vi "WF phase diversity_MATLAB_Correction_loop_AndorSDK_OneCorrApplyToAll.vi"() -> ()   [LabVIEW 2018]
uses:
  <userlib>/WaveKit.lib/Controls/Wavefront Corrector states - ONE.ctl
  <userlib>/WaveKit.lib/Classes/WavefrontCorrector/WavefrontCorrector.lvclass
  <userlib>/WaveKit.lib/Classes/WavefrontCorrectorSet/WavefrontCorrectorSet.lvclass
  <vilib>/Analysis/1siggen.llb/Ramp Pattern by Samples.vi
  <vilib>/Utility/file.llb/Read From Spreadsheet File (DBL).vi
  <vilib>/Analysis/1siggen.llb/Ramp Pattern by Delta.vi
  <vilib>/Analysis/NI_AALBase.lvlib
panel:
  in  "Tab Control":T1(tab)
  in  "Offset command file":path=path "D:/SystemAlignment/system_aberration_20200206.dat"
  in  "Initial haso file":path=path "D:/SystemAlignment/system_aberration_residual_20191015.has"
  out "# of Phase":i32
  in  "Error in":errorcluster
  in  "DM configuration file":path=path "C:/Program Files (x86)/Imagine Optic/Configuration Files/WaveFrontCorrector_mirao52-e_0326.dat"
  out "DM Initial State":T2[](array[typedef])
  out "DM ActuatorsNumber":i32
  out "Error out":errorcluster
  in  "EMCCD trigger port":tag="Dev1/port0/line0"
  in  "Cooler set to Temperature":i32=-60
  in  "Trigger":u32(ring)=1 items=["Internal", "External"]
  out "Return from CheckTimings":u32
  out "Calculated Exposure Value":sgl format="%.2f"
  out "Return from SetTemperature":u32
  out "Cooling":i32
  out "Return from Initialize":u32
  out "Detector X Pixels":i32
  out "Detector Y Pixels":i32
  in  "Initialize EMCCD?":bool=TRUE
  in  "Turn off EMCCD when finished?":bool=TRUE
  in  "Initial Zer coeff":dbl[](array[numeric])=[0.2, 0.2]
  in  "Initial Zer index":dbl[](array[numeric])=[4.0, 5.0]
  out "Initial Zer coeff\nRandomly generated":dbl[](array[numeric])
  out "Initial Zer index (starting from 4)\nrandomly generated":dbl[](array[numeric])
  in  "aberration tolerance":dbl=0.1 format="%#_13g"
  in  "aberration threshold":dbl=0.25 format="%#_13g"
  in  "?":enum16{"input manually ", "randomly generated"}(ring)
  in  "max random order":i64=9
  in  "NOT YET: Data Acquisition Iteration #":i32=1
  in  "Zern index in 2":i32[](array[numeric])=[3, 4, 5, 6, 7, 8]
  in  "Zern coef in 2":sgl[](array[numeric])=[0.0, 0.0, 0.2, 0.0, 0.0, 0.0]
  in  "Zern index in 3":i32[](array[numeric])=[3, 4, 5, 6, 7, 8]
  in  "Zern coef in 3":sgl[](array[numeric])=[0.2, 0.0, 0.0, 0.0, 0.0, 0.0]
  in  "Zern index in 4":i32[](array[numeric])=[3, 4, 5, 6, 7, 8]
  in  "Zern coef in 4":sgl[](array[numeric])=[0.2, 0.0, 0.0, 0.0, 0.0, 0.0]
  in  "Zern index in 5":i32[](array[numeric])=[3, 4, 5, 6, 7, 8]
  in  "Zern coef in 5":sgl[](array[numeric])=[0.0, 0.0, 0.0, 0.0, 0.0, -0.2]
  in  "Andor Picture/notes save to path":path=path "D:/YD/test/test1"
  in  "base name":string="beads_test"
  in  "Pics/phase":dbl=2.0
  in  "camera exposure time (s)":string="0.02"
  in  "# of Phase":i32=5
  in  "COMMAND matrix path":path=path "D:/SystemAlignment/IM_20200224.aomi"
  in  "488 shutter":refnum<k7>(container)
  in  "?":bool
  out "phase diversity file name":string
  out "Corrected Picture name":string
  in  "Z for correction (um) (10 steps=1um)":dbl format="%#_13g"
  in  "ASI stage VISA resource name":refnum<visa-resource-name>="COM5"
  in  "Z scanning range (um)":dbl format="%#_13g"
  in  "Z scanning step (um)":dbl format="%#_13g"
  out "Current Z in step":string="where z"
  in  "Use GPU":bool=TRUE
  in  "Show Recon":bool=TRUE
  in  "Show Input":bool
  in  "Background Value":u32=290
  in  "Crop Size of image":u32=512
  in  "Gamma Value":dbl=1e-06
  in  "Iteration Number":u32=10
  in  "Zernike Order":u32=15
  in  "Number for average":u32=2
  in  "Number of Phase":u32=2
  in  "Run MATLAB or correction?":bool=TRUE
  in  "Keep Reconstructed Defocus component?":bool
  # "If Pics/phase is 2:\npicture order:\n\noffset+aberr *2\nphase diversity *8\n\nground truth *1\noffset+aberr *1\ncorrected *2 but the last one cannot be seen in imagej"
  # "Randomly Generate Initial Zernike, enter here:"
  # "Manually input, enter here:"
  # "Andor Camera Settings"
  # "z-stack is from (Z_for_correction-Z_scanning_range) to (Z_for_correction+Z_scanning_range)"
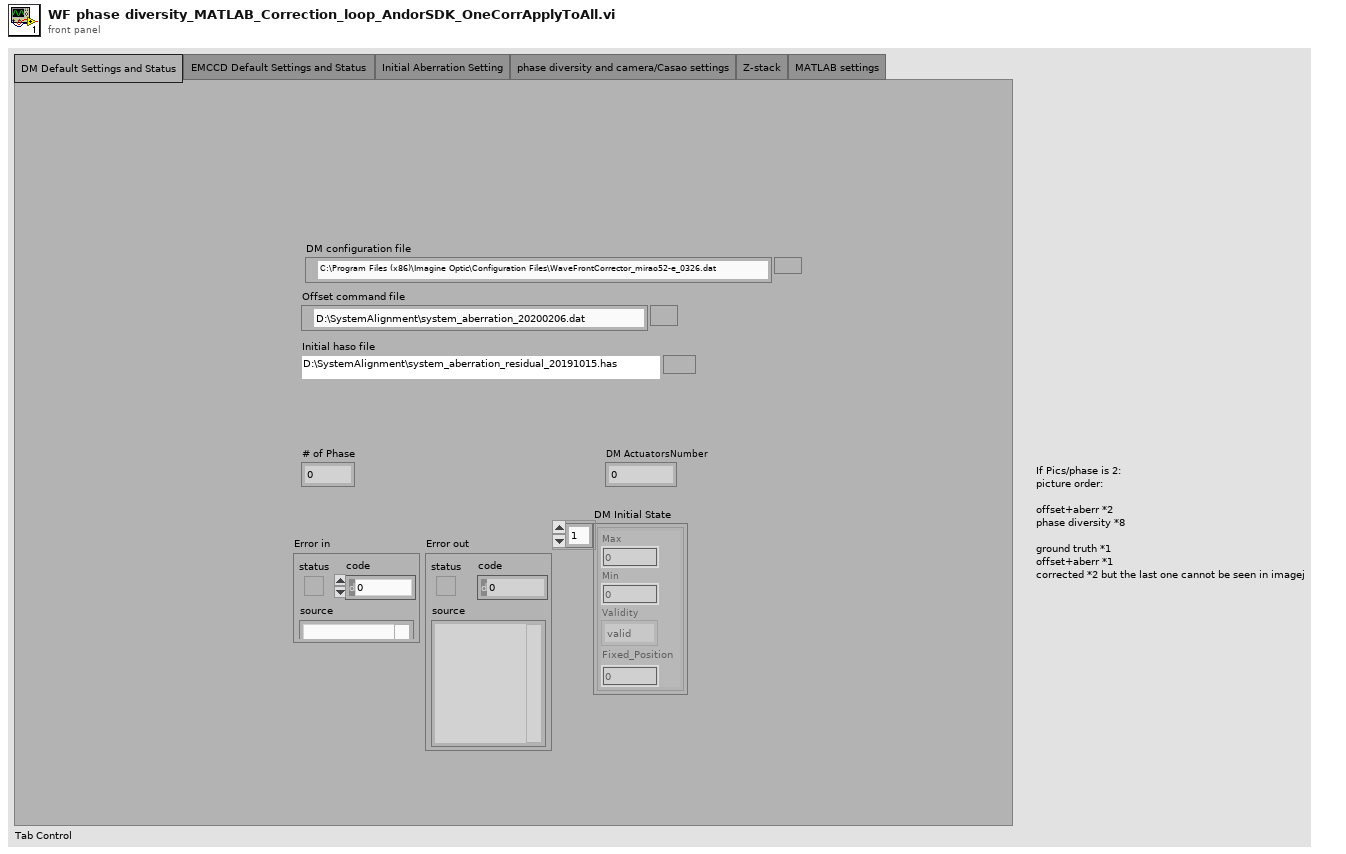
[diagram p1: front panel]
types:
  T1 = enum32{"DM Default Settings and Status", "EMCCD Default Settings and Status ", "Initial Aberration Setting", "phase diversity and camera/Casao settings", "Z-stack", "MATLAB settings"}
  T2 = typedef "Wavefront Corrector states - ONE.ctl" = cluster{"Max":sgl, "Min":sgl, "Validity":enum16{"valid", "fixed", "invalid"}, "Fixed_Position":sgl}
  T3 = typedef "Error Code Enum typedef.ctl" = enum32{"N/A (0)", "DRV_ERROR_CODES", "DRV_SUCCESS", "DRV_VXDNOTINSTALLED", "DRV_ERROR_SCAN", "DRV_ERROR_CHECK_SUM", "DRV_ERROR_FILELOAD", "DRV_UNKNOWN_FUNC", "DRV_ERROR_VXD_INIT", "DRV_ERROR_ADDRESS", "DRV_ERROR_PAGELOCK", "DRV_ERROR_PAGEUNLOCK", "DRV_ERROR_BOARDTEST", "DRV_ERROR_ACK", "DRV_ERROR_UP_FIFO", "DRV_ERROR_PATTERN", "N/A (16)", "DRV_ACQUISITION_ERRORS", "DRV_ACQ_BUFFER", "DRV_ACQ_DOWNFIFO_FULL", "DRV_PROC_UNKONWN_INSTRUCTION", "DRV_ILLEGAL_OP_CODE", "DRV_KINETIC_TIME_NOT_MET", "DRV_ACCUM_TIME_NOT_MET", "DRV_NO_NEW_DATA", "N/A (25)", "DRV_SPOOLERROR", "N/A (27)", "N/A (28)", "N/A (29)", "N/A (30)", "N/A (31)", "N/A (32)", "DRV_TEMPERATURE_CODES", "DRV_TEMPERATURE_OFF", "DRV_TEMPERATURE_NOT_STABILIZED", "DRV_TEMPERATURE_STABILIZED", "DRV_TEMPERATURE_NOT_REACHED", "DRV_TEMPERATURE_OUT_RANGE", "DRV_TEMPERATURE_NOT_SUPPORTED", "DRV_TEMPERATURE_DRIFT", "N/A (41)", "N/A (42)", "N/A (43)", "N/A (44)", "N/A (45)", "N/A (46)", "N/A (47)", "N/A (48)", "DRV_GENERAL_ERRORS", "DRV_INVALID_AUX", "DRV_COF_NOTLOADED", "DRV_FPGAPROG", "DRV_FLEXERROR", "DRV_GPIBERROR", "N/A (55)", "N/A (56)", "N/A (57)", "N/A (58)", "N/A (59)", "N/A (60)", "N/A (61)", "N/A (62)", "N/A (63)", "DRV_DATATYPE", "DRV_DRIVER_ERRORS", "DRV_P1INVALID", "DRV_P2INVALID", "DRV_P3INVALID", "DRV_P4INVALID", "DRV_INIERROR", "DRV_COFERROR", "DRV_ACQUIRING", "DRV_IDLE", "DRV_TEMPCYCLE", "DRV_NOT_INITIALIZED", "DRV_P5INVALID", "DRV_P6INVALID", "DRV_INVALID_MODE", "DRV_INVALID_FILTER", "DRV_I2CERRORS", "DRV_I2CDEVNOTFOUND", "DRV_I2CTIMEOUT", "DRV_P7INVALID", "N/A (84)", "N/A (85)", "N/A (86)", "N/A (87)", "N/A (88)", "N/A (89)", "DRV_IOCERROR", "DRV_VRMVERSIONERROR"}
  T4 = typedef "NI_Matrix.lvlib/RealMatrix.ctl" = dbl[][]
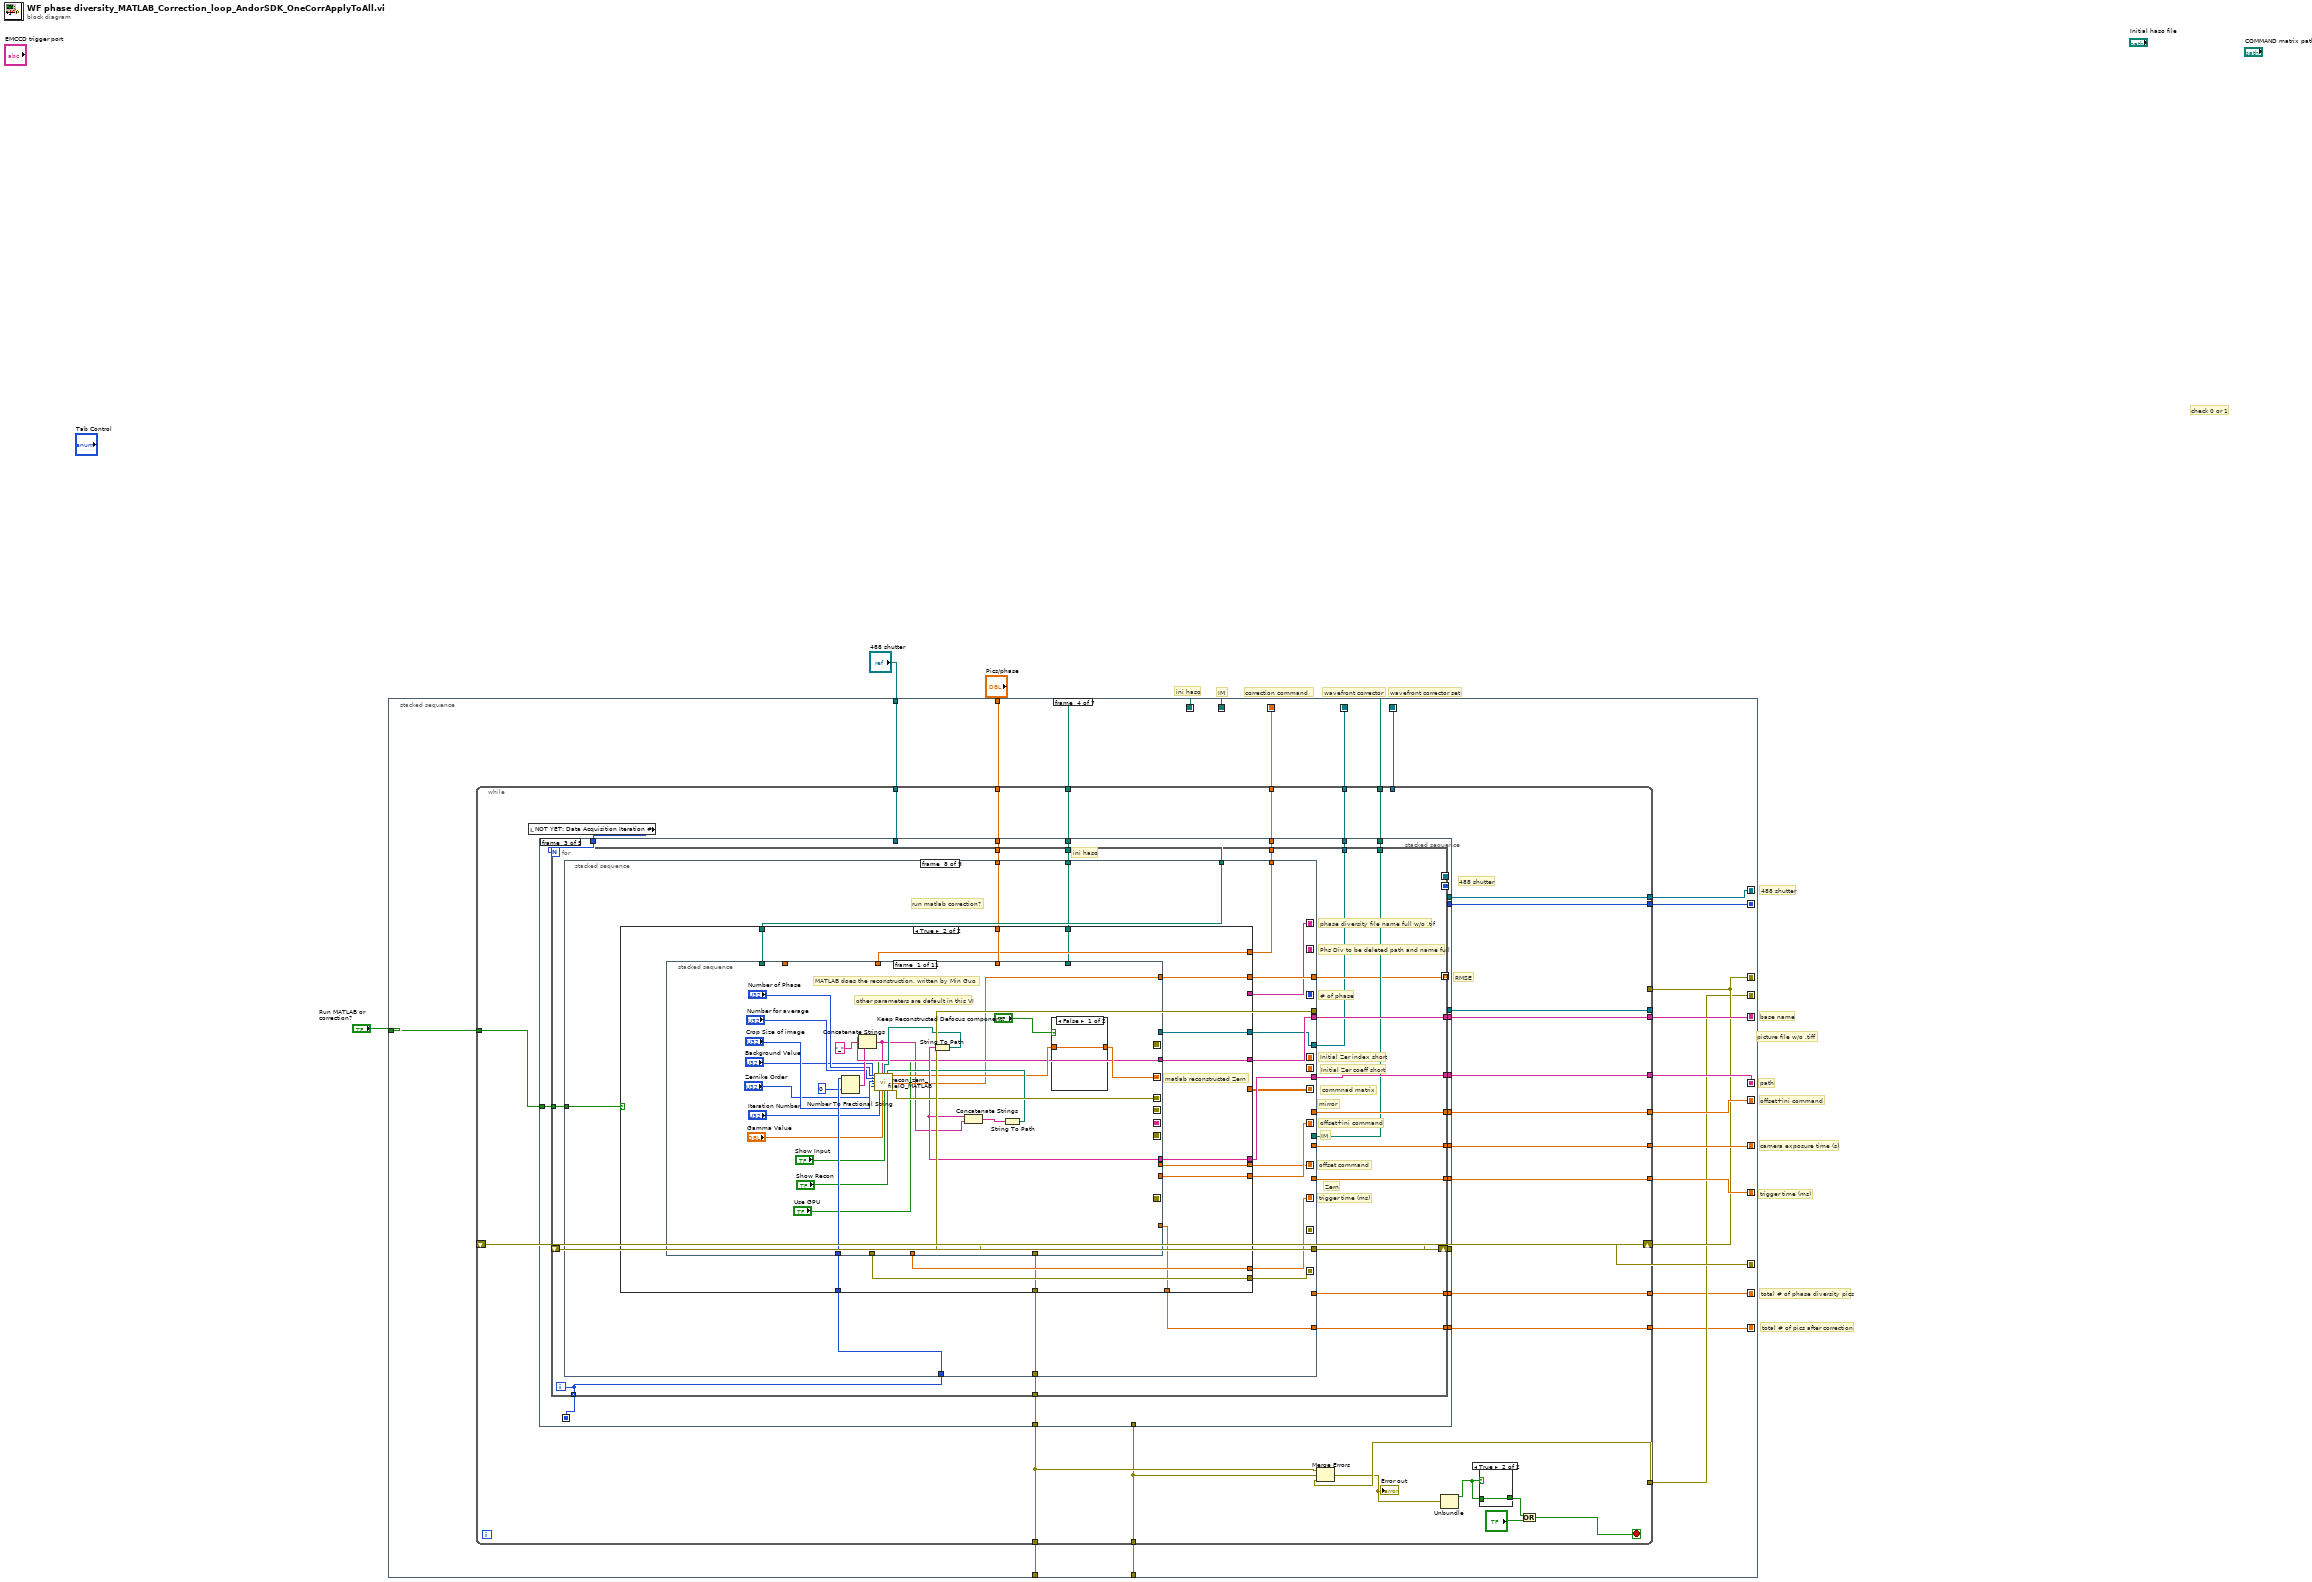
[diagram p0: block diagram]
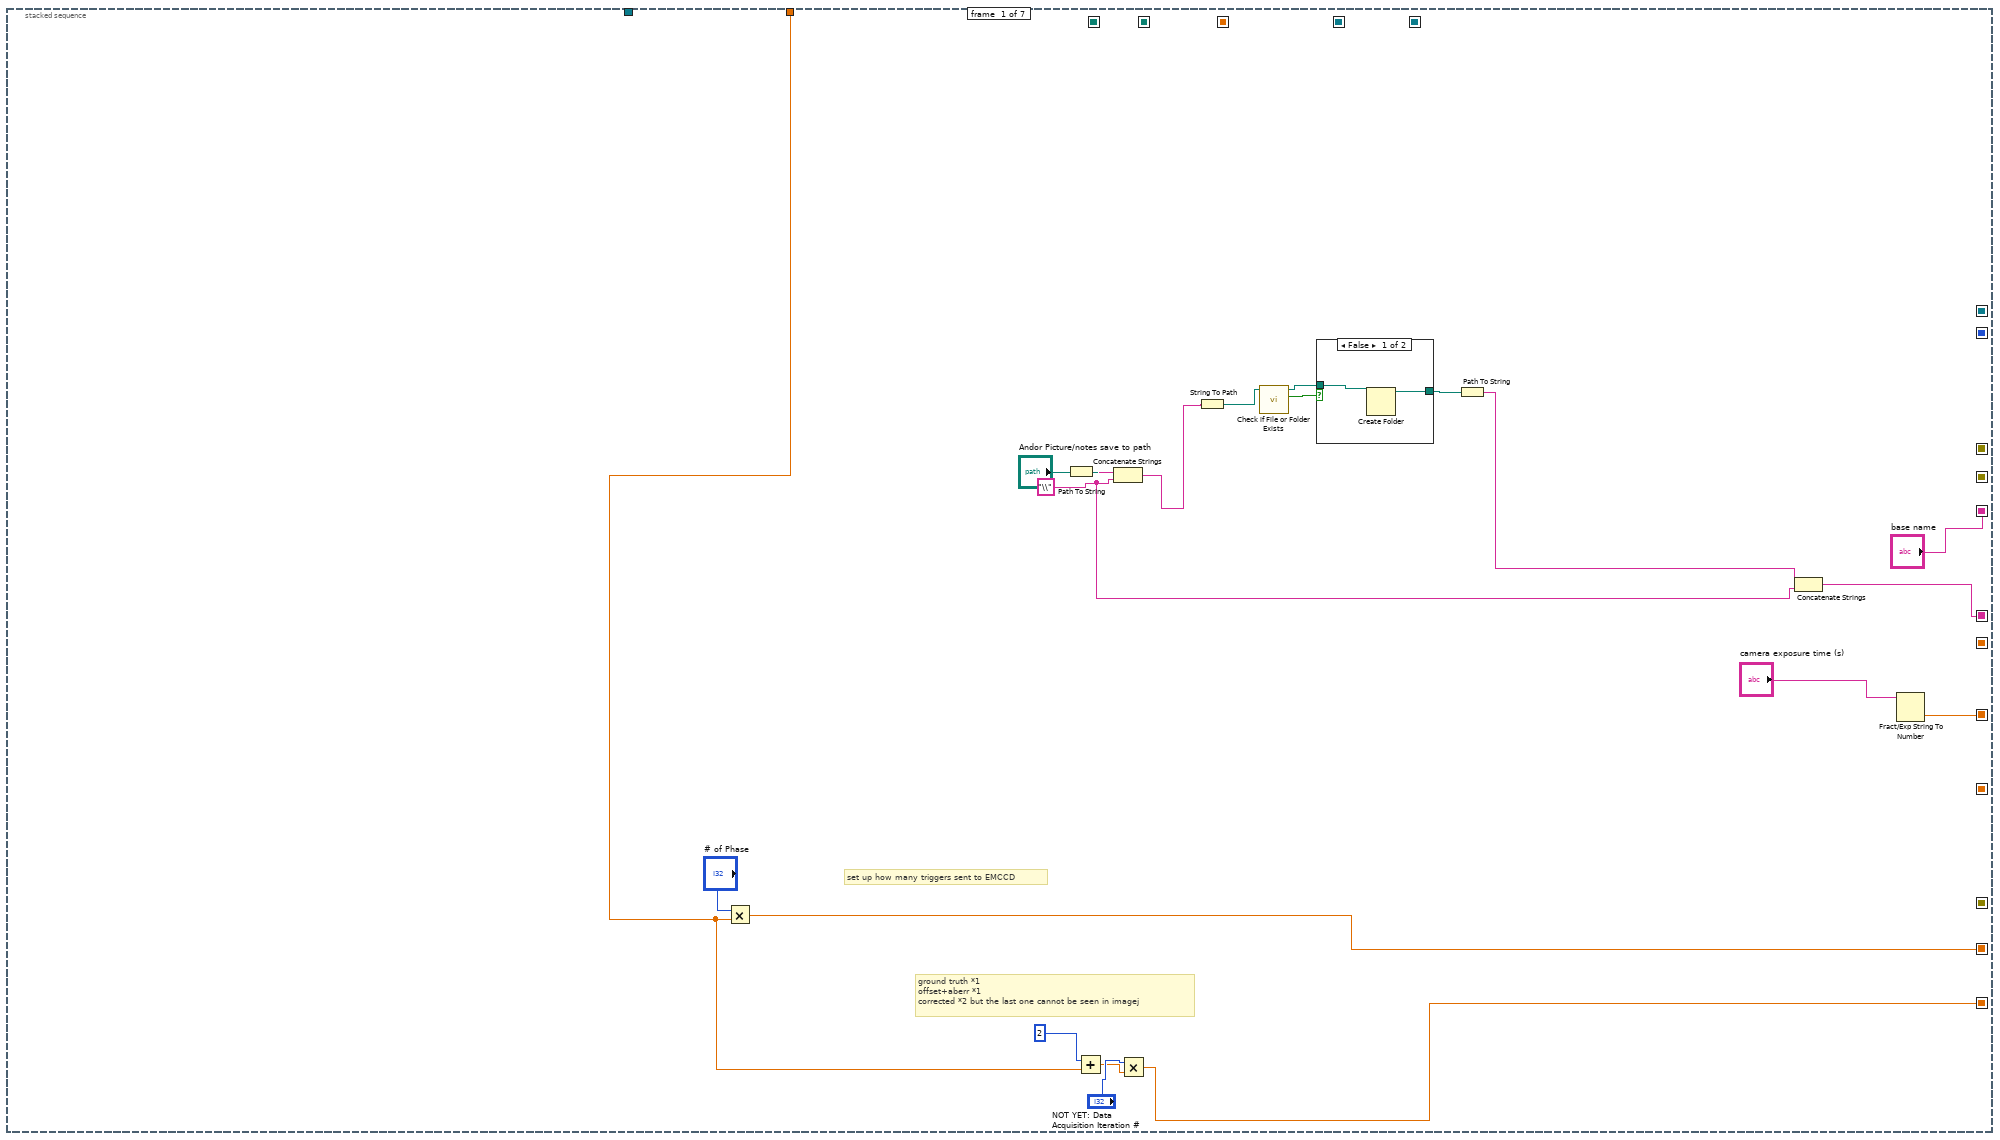
[diagram p2: hidden frame]
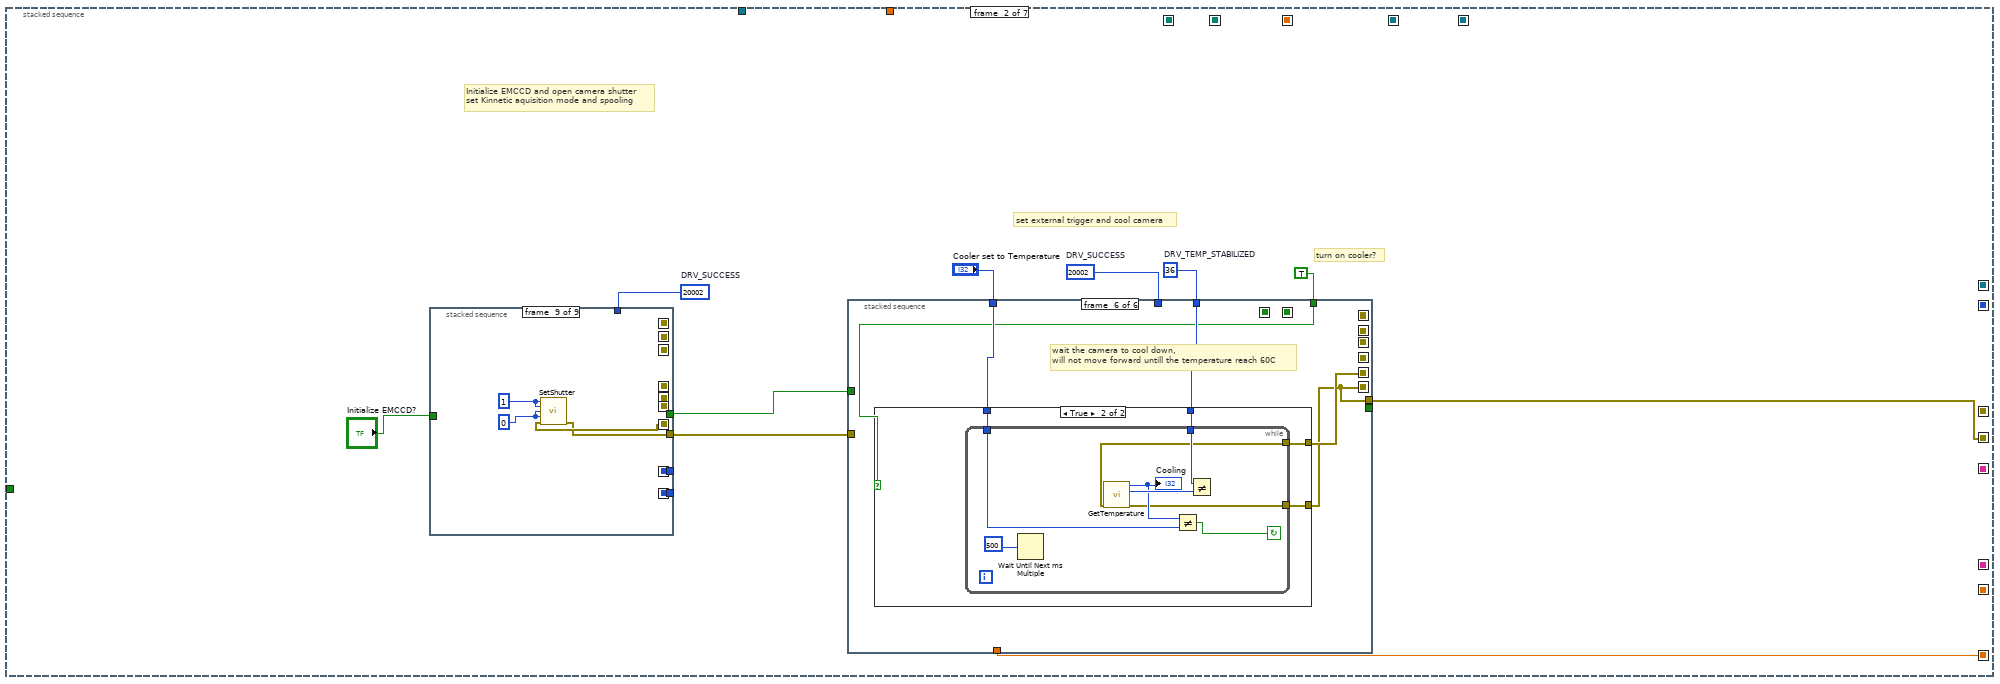
[diagram p4: hidden frame]
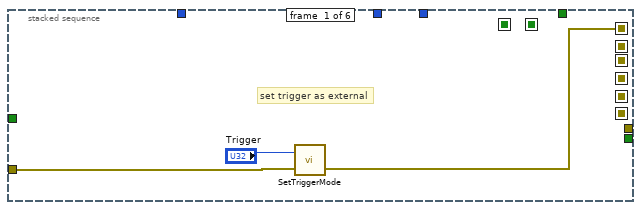
[diagram p5: hidden frame]
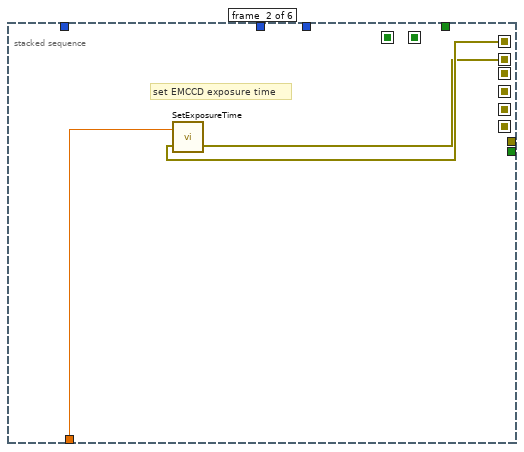
[diagram p6: hidden frame]
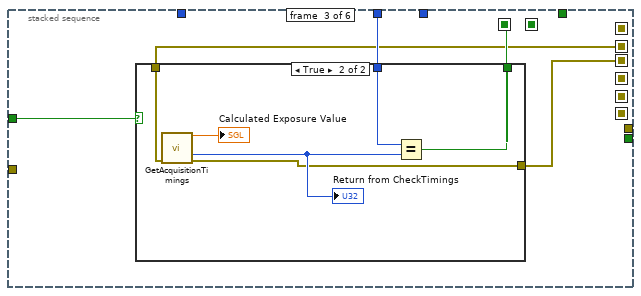
[diagram p7: hidden frame]
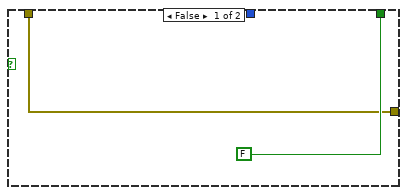
[diagram p8: hidden frame]
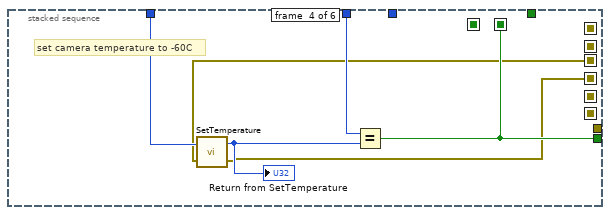
[diagram p9: hidden frame]
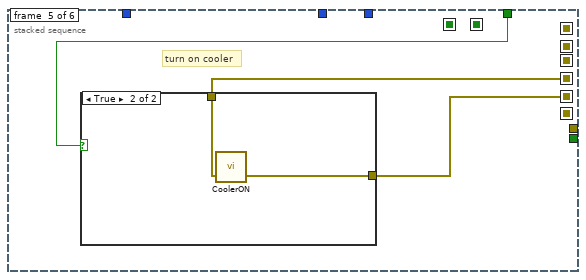
[diagram p10: hidden frame]
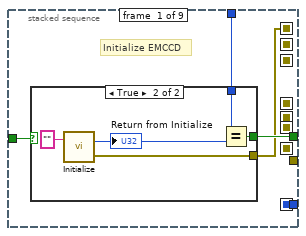
[diagram p13: hidden frame]
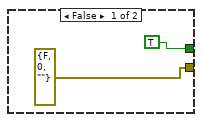
[diagram p14: hidden frame]
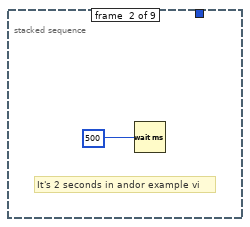
[diagram p15: hidden frame]
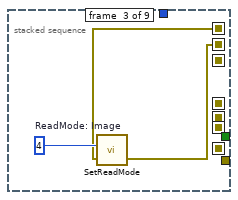
[diagram p16: hidden frame]
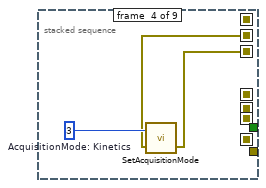
[diagram p17: hidden frame]
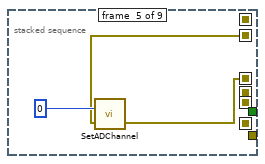
[diagram p18: hidden frame]
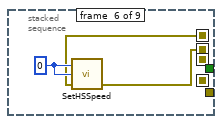
[diagram p19: hidden frame]
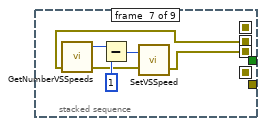
[diagram p20: hidden frame]
diagram:
  # "correction command"
  # "total # of phase diversity pics"
  # "picture file w/o .tiff"
  # "total # of pics after correction"
  # "wavefront corrector set"
  # "wavefront corrector"
  # "488 shutter"
  # "trigger time (ms)"
  # "offset+ini command"
  # "camera exposure time (s)"
  # "IM"
  # "ini haso"
  # "path"
  # "base name"
  # "check 0 or 1"
  n1 = stacked-sequence {
    seq-local: [w4 _ _ _ _ _ _] -> [_ _ _ w165 w632 _ _]
    seq-local: ["base name" _ _ _ _ _ _] -> [_ _ _ w164 w631 _ _]
    seq-local: [_ _ w144 _ _ _ _] -> [_ _ _ w163 _ _ _]
    seq-local: [_ _ w143 _ _ _ _] -> [_ _ _ w158 _ _ _]
    seq-local: [w18 _ _ _ _ _ _] -> [_ w29 _ w162 _ _ _]
    seq-local: [_ _ w128 _ _ _ _] -> [_ _ _ w150 _ _ _]
    seq-local: [_ _ _ w161 _ _ _] -> [_ _ _ _ _ _ _]
    seq-local: [_ _ _ w160 _ _ _] -> [_ _ _ _ w628 _ _]
    seq-local: [_ _ _ w159 _ _ _] -> [_ _ _ _ _ _ w714]
    seq-local: [_ _ _ w153 _ _ _] -> [_ _ _ _ w640 _ _]
    seq-local: [_ _ _ w156 _ _ _] -> [_ _ _ _ w639 _ _]
    seq-local: [_ _ w127 _ _ _ _] -> [_ _ _ w151 w637 _ w716]
    seq-local: [_ _ w126 _ _ _ _] -> [_ _ _ w149 _ _ w715]
    seq-local: [w15 _ _ _ _ _ _] -> [_ _ _ w146 _ _ _]
    seq-local: [_ w30 _ _ _ _ _] -> [_ _ _ w148 _ _ _]
    seq-local: [w14 _ _ _ _ _ _] -> [_ _ _ w147 _ _ _]
    seq-local: [_ _ _ w145 _ _ _] -> [_ _ _ _ w638 _ _]
    tunnel: "Pics/phase" -> [w12 _ _ w166 _ _ _]
    tunnel: "Run MATLAB or correction?" -> [_ _ _ w157 _ _ _]
    tunnel: [_ _ _ w155 _ _ _] -> _
    tunnel: [_ _ _ w154 _ _ _] -> _
    tunnel: "488 shutter" -> [_ _ _ w152 _ _ w717]
    frame #0 {
      w5 = "\\"
      # "set up how many triggers sent to EMCCD"
      # "ground truth *1\noffset+aberr *1\ncorrected *2 but the last one cannot be seen in imagej"
      n2 = Multiply(x="# of Phase", y=w12) -> (x*y=w14:dbl)
      n3 = Path To String(path="Andor Picture/notes save to path") -> (string=w20:string)
      n4 = Add(x=2, y=w12) -> (x+y=w16:dbl)
      n5 = Concatenate Strings(w20, w5) -> (w7:string)
      n6 = Multiply(x="NOT YET: Data Acquisition Iteration #", y=w16) -> (x*y=w15:dbl)
      n7 = String To Path(string=w7) -> (path=w11:path)
      n8 = call <vilib>:"Check if File or Folder Exists.vi"("path"=w11) -> ("file or folder exists?"=w9:bool, "dup path"=w10:path)  [unwired: 8 in, 1 out]
      n9 = case shown="False" w9 {
        tunnel: w10 -> [w25 w26]
        tunnel: [w24 w26] -> w8
        frame False {
          n10 = Create Folder(path (use dialog)=w25) -> (created path=w24:path)  [unwired: 2 in, 2 out]
        }
        frame True {
        }
      }
      n11 = Path To String(path=w8) -> (string=w6:string)
      n12 = Concatenate Strings(w6, w5) -> (w4:string)
      n13 = Fract/Exp String To Number(string="camera exposure time (s)") -> (number=w18:dbl)  [unwired: 3 in, 1 out]
    }
    frame #1 {
      w32 = 36  # DRV_TEMP_STABILIZED
      w34 = 20002  # DRV_SUCCESS
      w36 = 20002  # DRV_SUCCESS
      # "turn on cooler?"
      # "set external trigger and cool camera"
      # "Initialize EMCCD and open camera shutter\nset Kinnetic aquisition mode and spooling"
      n14 = stacked-sequence {
        seq-local: [_ _ _ _ _ _ _ w120 _] -> [_ _ _ _ _ _ _ _ _]
        seq-local: [_ _ _ _ _ _ _ w119 _] -> [_ _ _ _ _ _ _ _ _]
        seq-local: [w87 _ _ _ _ _ _ _ _] -> [_ _ w99 _ _ _ _ _ _]
        seq-local: [_ _ w98 _ _ _ _ _ _] -> [_ _ _ w102 _ _ _ _ _]
        seq-local: [_ _ _ w101 _ _ _ _ _] -> [_ _ _ _ w104 _ _ _ _]
        seq-local: [_ _ _ _ w105 _ _ _ _] -> [_ _ _ _ _ w108 _ _ _]
        seq-local: [_ _ _ _ _ w107 _ _ _] -> [_ _ _ _ _ _ w112 _ _]
        seq-local: [_ _ _ _ _ _ w110 _ _] -> [_ _ _ _ _ _ _ w118 _]
        seq-local: [_ _ _ _ _ _ _ w116 _] -> [_ _ _ _ _ _ _ _ w123]
        tunnel: w36 -> [w89 _ _ _ _ _ _ _ _]
        tunnel: [w88 _ _ _ _ _ _ _ _] -> w35
        tunnel: [_ _ _ _ _ _ _ w120 _] -> _
        tunnel: [_ _ _ _ _ _ _ w119 _] -> _
        tunnel: [_ _ _ _ _ _ _ _ w122] -> w31
        tunnel: "Initialize EMCCD?" -> [w86 _ _ _ _ _ _ _ _]
        frame #0 {
          # "Initialize EMCCD"
          n15 = case shown="True" w86 {
            tunnel: w89 -> [_ w94]
            tunnel: [TRUE w93] -> w88
            tunnel: [errorcluster {"status"=FALSE, "code"=0, "source"=""} ("Error in 2") w92] -> w87
            frame False {
            }
            frame True {
              n16 = call <userlib>:"Initialize.vi"("directory (\"\")"="" ("directory (\"\")")) -> ("error out"=w92:errorcluster, "DLL error code"=w96:u32)  [unwired: 1 in]
              "Return from Initialize" <- w96
              n17 = Equal?(x=w94, y=w96) -> (x = y?=w93:bool)
            }
          }
        }
        frame #1 {
          # "It's 2 seconds in andor example vi"
          n18 = Wait (ms)(milliseconds to wait=u32 500) -> ()  [unwired: 1 out]
        }
        frame #2 {
          w100 = u16 4  # ReadMode: Image
          n19 = call <userlib>:"SetReadMode.vi"("error in (no error)"=w99, "mode"=w100) -> ("error out"=w98:errorcluster)  [unwired: 1 out]
        }
        frame #3 {
          w103 = u16 3  # AcquisitionMode: Kinetics
          n20 = call <userlib>:"SetAcquisitionMode.vi"("error in (no error)"=w102, "mode"=w103) -> ("error out"=w101:errorcluster)  [unwired: 1 out]
        }
        frame #4 {
          n21 = call <userlib>:"SetADChannel.vi"("error in (no error)"=w104, "channel"=0) -> ("error out"=w105:errorcluster)  [unwired: 1 out]
        }
        frame #5 {
          w109 = 0
          n22 = call <userlib>:"SetHSSpeed.vi"("error in (no error)"=w108, "index"=w109, "type"=w109) -> ("error out"=w107:errorcluster)  [unwired: 1 in, 1 out]
        }
        frame #6 {
          n23 = call <userlib>:"GetNumberVSSpeeds.vi"("error in (no error)"=w112) -> ("error out"=w111:errorcluster, "number"=w115:i32)  [unwired: 2 in, 1 out]
          n24 = Subtract(x=w115, y=1) -> (x-y=w113:i32)
          n25 = call <userlib>:"SetVSSpeed.vi"("error in (no error)"=w111, "index"=w113) -> ("error out"=w110:errorcluster)  [unwired: 1 out]
        }
        frame #7 {
          w121 = 1
          n26 = call <userlib>:"GetDetector.vi"("error in (no error)"=w118) -> ("error out"=w117:errorcluster, "ypixels"=w120:i32, "xpixels"=w119:i32)  [unwired: 3 in, 1 out]
          "Detector Y Pixels" <- w120
          "Detector X Pixels" <- w119
          n27 = call <userlib>:"SetImage.vi"("hbin"=w121, "vbin"=w121, "hstart"=w121, "hend"=w119, "vstart"=w121, "vend"=w120, "error in (no error)"=w117) -> ("error out"=w116:errorcluster)  [unwired: 19 in, 1 out]
        }
        frame #8 {
          w124 = 0
          w125 = 1
          n28 = call <userlib>:"SetShutter.vi"("type"=w125, "mode"=w125, "closingtime"=w124, "openingtime"=w124, "error in (no error)"=w123) -> ("error out"=w122:errorcluster)  [unwired: 9 in, 1 out]
        }
      }
      n29 = stacked-sequence {
        seq-local: [_ _ w45 _ _ _] -> [_ _ _ _ _ _]
        seq-local: [_ _ _ w58 _ _] -> [_ _ _ _ _ _]
        seq-local: [w37 _ _ _ _ _] -> [_ w42 _ _ _ _]
        seq-local: [_ w41 _ _ _ _] -> [_ _ w44 _ _ _]
        seq-local: [_ _ w43 _ _ _] -> [_ _ _ w57 _ _]
        seq-local: [_ _ _ w56 _ _] -> [_ _ _ _ w64 _]
        seq-local: [_ _ _ _ w63 _] -> [_ _ _ _ _ w70]
        seq-local: [_ _ _ _ _ w68] -> [_ _ _ _ _ _]
        tunnel: w34 -> [_ _ w47 w61 _ _]
        tunnel: "Cooler set to Temperature" -> [_ _ _ w59 _ w71]
        tunnel: w32 -> [_ _ _ _ _ w72]
        tunnel: [_ _ _ w58 _ _] -> _
        tunnel: w35 -> [_ _ w46 _ _ _]
        tunnel: w31 -> [w38 _ _ _ _ _]
        tunnel: [_ _ _ _ _ w68] -> w30
        tunnel: w29 -> [_ w40 _ _ _ _]
        tunnel: TRUE -> [_ _ _ _ w62 w69]
        frame #0 {
          # "set trigger as external"
          n30 = call <userlib>:"SetTriggerMode.vi"("error in (no error)"=w38, "mode"="Trigger") -> ("error out"=w37:errorcluster)  [unwired: 1 out]
        }
        frame #1 {
          # "set EMCCD exposure time"
          n31 = call <userlib>:"SetExposureTime.vi"("error in (no error)"=w42, "time"=w40) -> ("error out"=w41:errorcluster)  [unwired: 1 out]
        }
        frame #2 {
          n32 = case shown="True" w46 {
            tunnel: w47 -> [_ w53]
            tunnel: [FALSE w55] -> w45
            tunnel: w44 -> [w48 w51]
            tunnel: [w48 w50] -> w43
            frame False {
            }
            frame True {
              n33 = call <userlib>:"GetAcquisitionTimings.vi"("error in (no error)"=w51) -> ("exposure"=→"Calculated Exposure Value":sgl, "DLL error code"=w52:u32, "error out"=w50:errorcluster)  [unwired: 10 in, 2 out]
              "Return from CheckTimings" <- w52
              n34 = Equal?(x=w53, y=w52) -> (x = y?=w55:bool)
            }
          }
        }
        frame #3 {
          # "set camera temperature to -60C"
          n35 = call <userlib>:"SetTemperature.vi"("error in (no error)"=w57, "temperature"=w59) -> ("error out"=w56:errorcluster, "DLL error code"=w60:u32)
          "Return from SetTemperature" <- w60
          n36 = Equal?(x=w61, y=w60) -> (x = y?=w58:bool)
        }
        frame #4 {
          # "turn on cooler"
          n37 = case shown="True" w62 {
            tunnel: w64 -> [w65 w67]
            tunnel: [w65 w66] -> w63
            frame False {
            }
            frame True {
              n38 = call <userlib>:"CoolerON.vi"("error in (no error)"=w67) -> ("error out"=w66:errorcluster)  [unwired: 1 in, 1 out]
            }
          }
        }
        frame #5 {
          # "wait the camera to cool down,\nwill not move forward untill the temperature reach 60C"
          n39 = case shown="True" w69 {
            tunnel: w72 -> [_ w77]
            tunnel: w71 -> [_ w76]
            tunnel: w70 -> [w73 w75]
            tunnel: [w73 w74] -> w68
            frame False {
            }
            frame True {
              n40 = while {
                tunnel: w77 -> [w84]
                tunnel: w76 -> [w81]
                tunnel: w75 -> [w79]
                tunnel: [w78] -> w74
                stop <- w80 continue-if-true
                n41 = Wait Until Next ms Multiple(millisecond multiple=u32 500) -> ()  [unwired: 1 out]
                n42 = call <userlib>:"GetTemperature.vi"("error in (no error)"=w79) -> ("error out"=w78:errorcluster, "status"=w83:T3, "temperature"=w82:i32)  [unwired: 3 in, 1 out]
                "Cooling" <- w82
                n43 = Not Equal?(x=w82, y=w81) -> (x != y?=w80:bool)
                n44 = Not Equal?(x=w84, y=w83) -> ()  [unwired: 1 out]
              }
            }
          }
        }
      }
    }
    frame #2 {
      # "Initialize CASAO"
      n45 = call <userlib>:"LVClass_WavefrontCorrectorSet ctor.vi"("WavefrontCorrectorSet in"=refnum<class "WavefrontCorrectorSet.lvclass"> refnum, "PathToWavefrontCorrectorSetupFile"="DM configuration file", "error in (no error)"="Error in") -> ("WavefrontCorrectorSet out"=w133:refnum<class "WavefrontCorrectorSet.lvclass">, "error out"=w142:errorcluster)  [unwired: 11 in]
      n46 = call <userlib>:"LVClass_WavefrontCorrector ctor.vi"("WavefrontCorrector in"=refnum<class "WavefrontCorrector.lvclass"> refnum, "PathToWavefrontCorrectorSetupFile"="DM configuration file", "error in (no error)"=w142) -> ("WavefrontCorrector out"=w137:refnum<class "WavefrontCorrector.lvclass">, "error out"=w136:errorcluster)  [unwired: 11 in]
      n47 = call <userlib>:"LVClass_WavefrontCorrector Init.vi"("WavefrontCorrector in"=w137, "set_init_state_from_config_file"=TRUE, "error in (no error)"=w136) -> ("WavefrontCorrector out"=w131:refnum<class "WavefrontCorrector.lvclass">, "error out"=w135:errorcluster)  [unwired: 11 in]
      n48 = call <userlib>:"LVClass_WavefrontCorrectorSet get nb of actuators.vi"("WavefrontCorrectorSet in"=w133, "error in (no error)"=w135) -> ("WavefrontCorrectorSet out"=w126:refnum<class "WavefrontCorrectorSet.lvclass">, "ActuatorsNumber"=→"DM ActuatorsNumber":i32, "error out"=w132:errorcluster)  [unwired: 11 in]
      n49 = call <userlib>:"LVClass_WavefrontCorrector Get Current Preferences.vi"("WavefrontCorrector in"=w131, "error in (no error)"=w132) -> ("WavefrontCorrector out"=w127:refnum<class "WavefrontCorrector.lvclass">, "Mirror preferences.Wavefront Corrector State"=→"DM Initial State":T2[], "error out"=w128:errorcluster)  [unwired: 10 in, 1 out]
      n50 = local read "COMMAND matrix path"() -> (w143:path)
      n51 = local read "Initial haso file"() -> (w144:path)
    }
    frame #3 {
      n52 = while {
        tunnel: w166 -> [w194]
        tunnel: w165 -> [w193]
        tunnel: w164 -> [w192]
        tunnel: w163 -> [w191]
        tunnel: w162 -> [w190]
        tunnel: [w188] -> w161
        tunnel: [w187] -> w160
        tunnel: w158 -> [w185]
        tunnel: w157 -> [w184]
        tunnel: [w183] -> w156
        tunnel: [w182] -> _
        tunnel: [w180] -> w155
        tunnel: [w181] -> w154
        shift-right: [w186] -> w159
        shift-left: w150 -> [w189]
        tunnel: [w179] -> w153
        tunnel: w152 -> [w178]
        tunnel: w151 -> [w177]
        tunnel: w150 -> [_]
        tunnel: w149 -> [_]
        tunnel: w148 -> [w175]
        tunnel: w147 -> [w169]
        tunnel: w146 -> [w168]
        tunnel: [w167] -> w145
        stop <- w171 stop-if-true
        # "488 shutter"
        # "RMSE"
        n53 = local read "NOT YET: Data Acquisition Iteration #"() -> (w176:i32)
        n54 = stacked-sequence {
          seq-local: [_ _ w218 _ _] -> [_ _ _ _ w623]
          seq-local: [_ _ w217 _ _] -> [_ _ _ _ _]
          seq-local: [_ w206 _ _ _] -> [_ _ _ w619 _]
          seq-local: [_ w207 _ _ _] -> [_ _ _ w618 _]
          tunnel: w194 -> [_ _ w230 _ _]
          tunnel: w193 -> [_ _ w229 _ w622]
          tunnel: w192 -> [_ _ w228 _ w621]
          tunnel: w191 -> [_ _ w227 _ _]
          tunnel: w190 -> [_ _ w226 _ _]
          tunnel: w189 -> [_ _ w225 _ _]
          tunnel: [_ _ w224 _ _] -> w188
          tunnel: [_ _ w223 _ _] -> w187
          tunnel: [_ _ w222 _ _] -> w186
          tunnel: w185 -> [_ _ w221 _ _]
          tunnel: w184 -> [_ _ w220 _ _]
          tunnel: w176 -> [_ _ w219 _ _]
          tunnel: [_ _ _ w617 _] -> w182
          tunnel: [_ _ _ w616 _] -> w183
          tunnel: [_ _ _ _ w620] -> w180
          tunnel: [_ _ w216 _ _] -> w181
          tunnel: [_ w206 _ _ _] -> w179
          tunnel: w178 -> [_ w205 _ _ _]
          tunnel: w177 -> [_ _ w215 _ _]
          tunnel: w169 -> [_ _ w214 _ _]
          tunnel: w168 -> [_ _ w213 _ _]
          tunnel: [_ _ w212 _ _] -> w167
          frame #0 {
            # "10 step=1um"
            # "MOVE TO Z FOR CORRECTION"
            n55 = Multiply(x="Z for correction (um) (10 steps=1um)", y=10.0) -> (x*y=w198:dbl)
            n56 = local read "ASI stage VISA resource name"() -> (w201:refnum<visa-resource-name>)
            n57 = Number To Decimal String(number=w198) -> (decimal integer string=w203:string)  [unwired: 1 in]
            n58 = Concatenate Strings("move z=", w203) -> (w202:string)
            n59 = call "WriteCmd.vi"("Command"=w202, "VISA resource name"=w201) -> ()  [unwired: 1 in, 1 out]
          }
          frame #1 {
            # "open the shutter of 488nm laser"
            n60 = property class="MG17Motor"(reference=w205, "HWSerialNum"=85819115.0) -> (reference out=w211:refnum<k7>)  [unwired: 1 in, 1 out]
            n61 = invoke class="MG17Motor" method="StartCtrl"(reference=w211) -> (reference out=w209:refnum<k7>)  [unwired: 2 in, 2 out]
            n62 = invoke class="MG17Motor" method="SC_Enable"(reference=w209, "lChanID"=0) -> (reference out=w206:refnum<k7>, "lChanID"=w207:i32)  [unwired: 2 in, 2 out]
          }
          frame #2 {
            n63 = for {
              N: w219 -> [_]
              tunnel: w230 -> [w248]
              tunnel: w229 -> [w247]
              tunnel: w228 -> [w246]
              tunnel: w227 -> [w245]
              tunnel: w226 -> [w244]
              tunnel: [w242] -> w224
              tunnel: [w241] -> w223
              tunnel: w221 -> [w239]
              tunnel: w220 -> [w238]
              shift-right: [w240] -> w222
              shift-left: w225 -> [w243]
              tunnel: [w237] -> w218 mode=indexing
              tunnel: [w236] -> w217 mode=indexing
              tunnel: [w235] -> w216
              tunnel: w215 -> [w234]
              tunnel: w214 -> [w233]
              tunnel: w213 -> [w232]
              tunnel: [w231] -> w212
              i -> [w236]
              # "Phs Div to be deleted path and name full"
              # "phase diversity file name full w/o .tif"
              # "# of phase"
              # "trigger time (ms)"
              # "offset+ini command"
              # "Initial Zer coeff short"
              # "Initial Zer index short"
              # "mirror"
              # "Zern"
              # "commnad matrix"
              # "ini haso"
              # "IM"
              # "offset command"
              n64 = stacked-sequence {
                seq-local: [_ w260 _ _ _ _ _ _ _] -> [_ _ w280 _ w408 _ _ w463 _]
                seq-local: [_ _ w278 _ _ _ _ _ _] -> [_ _ _ _ w407 _ _ w465 _]
                seq-local: [_ _ w276 _ _ _ _ _ _] -> [_ _ _ _ w406 _ _ _ _]
                seq-local: [_ _ w269 _ _ _ _ _ _] -> [_ _ _ _ w403 _ _ _ _]
                seq-local: [w251 _ _ _ _ _ _ _ _] -> [_ _ w266 _ _ _ _ _ _]
                seq-local: [w250 _ _ _ _ _ _ _ _] -> [_ _ w265 _ _ _ _ _ _]
                seq-local: [_ _ w264 _ _ _ _ _ _] -> [_ _ _ _ _ _ _ w471 _]
                seq-local: [_ _ _ _ w402 _ _ _ _] -> [_ _ _ _ _ w443 _ w469 _]
                seq-local: [_ _ _ _ w401 _ _ _ _] -> [_ _ _ _ _ _ _ w468 _]
                seq-local: [_ _ _ _ _ _ w446 _ _] -> [_ _ _ _ _ _ _ w459 _]
                seq-local: [_ _ _ w395 _ _ _ _ _] -> [_ _ _ _ _ _ _ _ w605]
                tunnel: w248 -> [_ _ w273 _ w411 _ _ w470 _]
                tunnel: w247 -> [_ _ w274 w398 w410 _ w454 w473 _]
                tunnel: w246 -> [_ _ w275 w397 w409 _ w456 w474 _]
                tunnel: w245 -> [_ _ w272 _ _ _ _ w457 _]
                tunnel: w239 -> [_ _ w271 _ w405 _ _ _ _]
                tunnel: w244 -> [_ _ _ _ w404 _ _ _ _]
                tunnel: w243 -> [_ _ w270 _ _ _ _ _ _]
                tunnel: [_ _ _ _ w401 _ _ _ _] -> w240
                tunnel: [_ _ w264 _ _ _ _ _ _] -> w242
                tunnel: [_ _ _ _ w402 _ _ _ _] -> w241
                tunnel: w239 -> [_ _ _ _ _ _ _ w472 _]
                tunnel: w238 -> [_ _ _ _ _ _ _ w467 _]
                tunnel: w236 -> [_ _ w263 w394 _ _ w455 w466 _]
                tunnel: [_ _ _ _ _ _ _ w464 _] -> w237
                tunnel: [_ _ _ _ _ _ _ w462 _] -> w235
                tunnel: w234 -> [_ _ _ _ w400 _ _ w461 _]
                tunnel: w233 -> [_ _ _ w399 _ _ _ _ w603]
                tunnel: w232 -> [_ _ _ _ _ _ _ w460 _]
                tunnel: [_ _ _ _ _ _ _ w458 _] -> w231
                frame #0 {
                  # "generate initial aberration (aberr to correct)"
                  n65 = case shown="\"randomly generated\"" "?" {
                    tunnel: ["Initial Zer index" w257] -> w251
                    tunnel: ["Initial Zer coeff" w256] -> w250
                    tunnel: "max random order" -> [_ w255]
                    frame "input manually " {
                    }
                    frame "randomly generated" {
                      # "generate random zernike index and coefficient arrays"
                      n66 = call "Random Aberration Array Generator.vi"("max random order"=w255, "aberration tolerance"="aberration tolerance", "aberration threshold"="aberration threshold") -> ("Zer coeff"=w256:dbl[], "Zer index (starting from 3)"=w257:dbl[])  [unwired: 7 in]
                      "Initial Zer index (starting from 4)\nrandomly generated" <- w257
                      "Initial Zer coeff\nRandomly generated" <- w256
                    }
                  }
                }
                frame #1 {
                  # "read in offset command"
                  n67 = call-poly <vilib>:"Read From Spreadsheet File.vi"("format (%.3f)"="%.8f", "file path (dialog if empty)"="Offset command file") -> ("first row"=w260:dbl[])  [unwired: 5 in, 4 out]
                }
                frame #2 {
                  w285 = 0.0
                  # "ini zern coeff"
                  # "offset+ini command"
                  # "Zern coeff"
                  # "Zern index"
                  # "calculate the command:\nfor phase diversity"
                  n68 = Array Size(array="Zern index in 2") -> (size(s)=w283:i32)
                  n69 = call-poly <vilib>:"Ramp Pattern.vi"("start"=w285, "end"=w285, "samples"=w283) -> ("Ramp Pattern"=w282:dbl[])  [unwired: 7 in, 1 out]
                  n70 = Build Array(w282, "Zern index in 2", "Zern index in 3", "Zern index in 4", "Zern index in 5") -> (w267:T4)
                  n71 = Build Array(w282, "Zern coef in 2", "Zern coef in 3", "Zern coef in 4", "Zern coef in 5") -> (w286:T4)
                  n72 = Transpose Matrix(1:w286) -> (0:w279:T4)
                  n73 = Transpose Matrix(1:w267) -> (0:w277:T4)
                  n74 = Array Size(array=w267) -> (size(s)=w268:i32[])
                  n75 = Index Array(array=w268, index=1) -> (element=w276:i32)
                  "# of Phase" <- w276
                  n76 = stacked-sequence {
                    seq-local: [w295 _ _] -> [_ w313 w379]
                    seq-local: [w296 _ _] -> [_ w307 _]
                    seq-local: [_ w306 _] -> [_ _ w376]
                    seq-local: [w294 _ _] -> [_ w305 _]
                    tunnel: w276 -> [_ w318 _]
                    tunnel: w266 -> [w303 _ _]
                    tunnel: w265 -> [w302 w308 _]
                    tunnel: w271 -> [w301 w315 _]
                    tunnel: w280 -> [w299 _ _]
                    tunnel: w277 -> [_ w317 _]
                    tunnel: w279 -> [_ w316 _]
                    tunnel: w272 -> [w298 w314 _]
                    tunnel: [_ w312 _] -> w278
                    tunnel: w275 -> [_ w310 w377]
                    tunnel: w274 -> [_ w311 w378]
                    tunnel: w273 -> [_ w309 _]
                    tunnel: w270 -> [w297 _ _]
                    tunnel: [_ _ w375] -> w269
                    tunnel: [w295 _ _] -> w264
                    tunnel: w263 -> [_ w304 w373]
                    frame #0 {
                      n77 = call "zern2command_test.vi"("Initial haso file"=w298, "error in (no error)"=w297, "interaction matrix file"=w301, "Zern coef in"=w302, "Zern index in"=w303) -> ("error out"=w296:errorcluster, "Zern coef out"=w294:sgl[], "Offset positions"=w300:sgl[])  [unwired: 4 in]
                      n78 = Add(x=w300, y=w299) -> (x+y=w295:dbl[])
                    }
                    frame #1 {
                      n79 = for {
                        N: w318 -> [w321]
                        tunnel: w317 -> [w334] mode=indexing
                        tunnel: w316 -> [w333] mode=indexing
                        tunnel: w315 -> [w332]
                        tunnel: w314 -> [w331]
                        tunnel: w313 -> [w330]
                        tunnel: [w329] -> w312 mode=indexing
                        tunnel: w311 -> [w328]
                        tunnel: w310 -> [w327]
                        tunnel: w309 -> [w326]
                        tunnel: w308 -> [w325]
                        tunnel: w307 -> [w324]
                        tunnel: [w323] -> w306
                        tunnel: w305 -> [w320]
                        tunnel: w304 -> [w319]
                        i -> [w322]
                        n80 = stacked-sequence {
                          seq-local: [w340 _] -> [_ w359]
                          seq-local: [w336 _] -> [_ w358]
                          tunnel: w334 -> [w349 _]
                          tunnel: w333 -> [w348 _]
                          tunnel: w332 -> [w347 _]
                          tunnel: w331 -> [w346 _]
                          tunnel: w330 -> [w344 _]
                          tunnel: [w343 _] -> w329
                          tunnel: w328 -> [_ w361]
                          tunnel: w327 -> [_ w360]
                          tunnel: w326 -> [_ _]
                          tunnel: w322 -> [w342 _]
                          tunnel: w325 -> [w338 _]
                          tunnel: w324 -> [w337 _]
                          tunnel: [_ w357] -> w323
                          tunnel: w322 -> [_ _]
                          tunnel: w321 -> [_ _]
                          tunnel: w320 -> [w335 _]
                          tunnel: w319 -> [_ w354]
                          frame #0 {
                            n81 = Equal To 0?(x=w342) -> (x = 0?=w341:bool)
                            n82 = call "zern2command_test.vi"("Initial haso file"=w346, "error in (no error)"=w337, "interaction matrix file"=w347, "Zern coef in"=w348, "Zern index in"=w349) -> ("error out"=w336:errorcluster, "Zern coef out"=w339:sgl[], "Offset positions"=w345:sgl[])  [unwired: 4 in]
                            n83 = case shown="False" w341 {
                              tunnel: [w350 w351] -> w340
                              tunnel: w339 -> [w350 _]
                              tunnel: w338 -> [_ _]
                              tunnel: w335 -> [_ w351]
                              frame False {
                              }
                              frame True {
                              }
                            }
                            n84 = Add(x=w344, y=w345) -> (x+y=w343:dbl[])
                          }
                          frame #1 {
                            n85 = Number To Fractional String(number=w354, precision (6)=0) -> (F-format string=w353:string)  [unwired: 2 in]
                            n86 = Concatenate Strings(w361, w360, "_", w353, "_coeff.txt") -> (w369:string)
                            n87 = String To Path(string=w369) -> (path=w368:path)
                            n88 = Open/Create/Replace File(file path (use dialog)=w368, error in=w358, operation (0:open)=3) -> (refnum out=w365:refnum<file>, error out=w366:errorcluster)  [unwired: 3 in, 1 out]
                            n89 = Array To Spreadsheet String(array=w359, 3:"%f") -> (spreadsheet string=w356:string)  [unwired: 1 in]
                            n90 = Set File Position(refnum=w365, from (0:start)=1, error in=w366) -> (refnum out=w363:refnum<file>, error out=w362:errorcluster)  [unwired: 1 in]
                            n91 = Write to Text File(file (use dialog)=w363, text=w356, error in=w362) -> (error out=w357:errorcluster)  [unwired: 1 in, 2 out]
                          }
                        }
                      }
                    }
                    frame #2 {
                      n92 = Number To Fractional String(number=w373, precision (6)=0) -> (F-format string=w372:string)  [unwired: 2 in]
                      n93 = Concatenate Strings(w378, w377, "_", w372, "_IniAbr+offset.txt") -> (w388:string)
                      n94 = String To Path(string=w388) -> (path=w386:path)
                      n95 = Open/Create/Replace File(file path (use dialog)=w386, error in=w376, operation (0:open)=3) -> (refnum out=w383:refnum<file>, error out=w384:errorcluster)  [unwired: 3 in, 1 out]
                      n96 = Array To Spreadsheet String(array=w379, 3:"%f") -> (spreadsheet string=w390:string)  [unwired: 1 in]
                      n97 = Set File Position(refnum=w383, from (0:start)=1, error in=w384) -> (refnum out=w381:refnum<file>, error out=w380:errorcluster)  [unwired: 1 in]
                      n98 = Write to Text File(file (use dialog)=w381, text=w390, error in=w380) -> (error out=w375:errorcluster)  [unwired: 1 in, 2 out]
                    }
                  }
                }
                frame #3 {
                  # "set andor kinetics and spooling, \nstart acquire and wait for the external trigger"
                  n99 = Number To Fractional String(number=w394, precision (6)=0) -> (F-format string=w392:string)  [unwired: 2 in]
                  n100 = Concatenate Strings(w398, w397, "_PhsDiv_ToBeDeleted_", w392) -> (w395:string)
                  n101 = call "SetSpool_WaitForExtTrigger.vi"("path and name"=w395, "Kinetic Series"=w399) -> ()  [unwired: 10 in]
                }
                frame #4 {
                  # "take phase diversity pictures"
                  n102 = for {
                    N: w406 -> [_]
                    tunnel: w411 -> [w422]
                    tunnel: w410 -> [w421]
                    tunnel: w409 -> [w420]
                    tunnel: w405 -> [w419]
                    tunnel: w408 -> [w418]
                    tunnel: w407 -> [w417] mode=indexing
                    tunnel: w404 -> [w416]
                    tunnel: w403 -> [w415]
                    tunnel: [w414] -> w401
                    tunnel: [w413] -> w402
                    tunnel: w400 -> [w412]
                    n103 = stacked-sequence {
                      seq-local: [w423 _] -> [_ w432]
                      tunnel: w422 -> [_ w434]
                      tunnel: w421 -> [_ _]
                      tunnel: w420 -> [_ _]
                      tunnel: w419 -> [_ _]
                      tunnel: w418 -> [_ _]
                      tunnel: w417 -> [w424 _]
                      tunnel: w416 -> [_ w433]
                      tunnel: w415 -> [w425 _]
                      tunnel: [_ w431] -> w414
                      tunnel: [_ w430] -> w413
                      tunnel: w412 -> [w426 _]
                      frame #0 {
                        # "response time of mirror"
                        n104 = call <userlib>:"LVClass_WavefrontCorrector Move to Absolute Position.vi"("WavefrontCorrector in"=w426, "Absolute Positions"=w424, "error in (no error)"=w425) -> ("error out"=w423:errorcluster)  [unwired: 11 in, 1 out]
                        n105 = Add(x=5, y=10) -> (x+y=w427:i32)
                        n106 = Wait (ms)(milliseconds to wait=w427) -> ()  [unwired: 1 out]
                      }
                      frame #1 {
                        n107 = for {
                          N: w434 -> [_]
                          tunnel: w433 -> [w439]
                          tunnel: w432 -> [w437]
                          tunnel: [w436] -> w431
                          tunnel: [w435] -> w430
                          n108 = local read "EMCCD trigger port"() -> (w442:tag)
                          n109 = Add(x=w439, y=0.04) -> (x+y=w438:dbl)
                          n110 = Multiply(x=w438, y=1000.0) -> (x*y=w435:dbl)
                          n111 = call "trig EMCCD.vi"("error in (no error)"=w437, "exp time (ms)"=w435, "lines"=w442) -> ("error out"=w436:errorcluster)
                        }
                      }
                    }
                  }
                }
                frame #5 {
                  # "send out a trigger to EMCCD to end the aquisition."
                  n112 = local read "EMCCD trigger port"() -> (w444:tag)
                  n113 = call "trig EMCCD.vi"("exp time (ms)"=w443, "lines"=w444) -> ()  [unwired: 1 in, 1 out]
                }
                frame #6 {
                  w451 = 0
                  # "save phase diversity pictures:\npictures per phase*number of phases (Eg: 2*5=10 pictures in this file)"
                  n114 = Number To Fractional String(number=w455, precision (6)=w451) -> (F-format string=w450:string)  [unwired: 2 in]
                  n115 = Concatenate Strings(w456, "_", w450) -> (w446:string)
                  "phase diversity file name" <- w446
                  n116 = Concatenate Strings(w446, ".tif") -> (w447:string)
                  n117 = Concatenate Strings(w454, w447) -> (w449:string)
                  n118 = call <userlib>:"SaveAsTiff.vi"("path"=w449, "palette"="C:\\Program Files\\Andor SOLIS\\GREY.PAL", "position"=w451, "type"=1) -> ()  [unwired: 10 in, 2 out]
                }
                frame #7 {
                  # "run matlab correction?"
                  n119 = case shown="True" w467 {
                    tunnel: w473 -> [_ w492]
                    tunnel: w474 -> [_ w491]
                    tunnel: w472 -> [_ w490]
                    tunnel: w471 -> [w475 w489]
                    tunnel: w469 -> [_ w488]
                    tunnel: w470 -> [_ w487]
                    tunnel: w468 -> [_ w486]
                    tunnel: w466 -> [_ w485]
                    tunnel: w465 -> [_ _]
                    tunnel: [0 w484] -> w464
                    tunnel: w463 -> [_ w483]
                    tunnel: [errorcluster {"status"=FALSE, "code"=0, "source"=""} ("Error out 2") w482] -> w462
                    tunnel: w461 -> [_ w481]
                    tunnel: w460 -> [_ w480]
                    tunnel: w459 -> [_ _]
                    tunnel: [w475 w479] -> w458
                    tunnel: w457 -> [_ w478]
                    frame False {
                    }
                    frame True {
                      # "matlab reconstructed Zern"
                      n120 = stacked-sequence {
                        seq-local: [w510 _ _ _ _ _ _ _ _ _ _] -> [_ _ _ _ _ _ w565 _ _ _ _]
                        seq-local: [w516 _ _ _ _ _ _ _ _ _ _] -> [_ _ _ _ _ _ w561 _ _ _ _]
                        seq-local: [_ _ _ _ w543 _ _ _ _ _ _] -> [_ _ _ _ _ w550 _ _ _ _ _]
                        seq-local: [_ _ w531 _ _ _ _ _ _ _ _] -> [_ _ _ w538 _ _ _ _ _ _ _]
                        seq-local: [_ _ _ w540 _ _ _ _ _ _ _] -> [_ _ _ _ w544 _ _ _ _ _ _]
                        seq-local: [_ w523 _ _ _ _ _ _ _ _ _] -> [_ _ _ _ _ _ _ _ _ _ w592]
                        seq-local: [_ _ _ _ _ _ w555 _ _ _ _] -> [_ _ _ _ _ _ _ w570 _ _ _]
                        tunnel: w492 -> [w515 w526 _ _ _ _ _ _ _ w581 _]
                        tunnel: w491 -> [w509 w525 _ _ _ _ _ _ _ w580 _]
                        tunnel: w490 -> [_ _ _ _ _ _ w564 _ _ _ _]
                        tunnel: w489 -> [_ _ _ _ w545 _ w563 _ _ _ _]
                        tunnel: w488 -> [_ _ _ w542 _ w552 _ w572 w578 _ _]
                        tunnel: w486 -> [_ _ w532 _ _ _ _ _ _ _ _]
                        tunnel: [_ _ _ w541 _ _ _ _ _ _ _] -> _
                        tunnel: w487 -> [_ _ _ w541 _ _ _ w571 _ _ _]
                        tunnel: w485 -> [w507 w524 _ _ _ _ _ _ _ w582 _]
                        tunnel: [w494 _ _ _ _ _ _ _ _ _ _] -> w484
                        tunnel: w483 -> [_ _ w533 _ _ _ _ _ _ _ _]
                        tunnel: [_ _ _ _ _ _ _ w569 _ _ _] -> w482
                        tunnel: w481 -> [_ _ w534 _ w546 _ w557 _ _ _ _]
                        tunnel: w480 -> [_ w527 _ _ _ _ _ _ _ _ w590]
                        tunnel: [_ _ _ _ _ _ w554 _ _ _ _] -> w479
                        tunnel: w478 -> [_ _ _ _ _ _ w553 _ _ _ _]
                        frame #0 {
                          # "MATLAB does the reconstruction, written by Min Guo"
                          # "other parameters are default in this VI"
                          n121 = Number To Fractional String(number=w507, precision (6)=0) -> (F-format string=w505:string)  [unwired: 2 in]
                          n122 = Concatenate Strings(w509, "_", w505) -> (w493:string)
                          n123 = String To Path(string=w515) -> (path=w517:path)
                          n124 = Concatenate Strings(w515, w493) -> (w514:string)
                          n125 = String To Path(string=w514) -> (path=w513:path)
                          n126 = call "recon_zern_fileIO_MATLAB.vi"("Number of Phase"="Number of Phase", "Number for average"="Number for average", "Crop Size of image"="Crop Size of image", "Background Value"="Background Value", "Zernike Order"="Zernike Order", "Use GPU"="Use GPU", "Iteration Number"="Iteration Number", "File Name"=w493, "Gamma Value"="Gamma Value", "Path In"=w517, "Show Input"="Show Input", "Path Out"=w513, "Show Recon"="Show Recon") -> ("Zern coef out"=w511:sgl[], "RMSE Value"=w494:dbl, "error out"=w516:errorcluster)  [unwired: 3 in, 1 out]
                          n127 = case shown="False" "Keep Reconstructed Defocus component?" {
                            tunnel: w511 -> [w518 w522]
                            tunnel: [w518 w519] -> w510
                            frame False {
                            }
                            frame True {
                              n128 = Replace Array Subset(array=w522, new element=0.0, index=2) -> (w519:sgl[])
                            }
                          }
                        }
                        frame #1 {
                          # "set andor kinetics and spooling, \nstart acquire and wait for the external trigger"
                          n129 = Number To Fractional String(number=w524, precision (6)=0) -> (F-format string=w528:string)  [unwired: 2 in]
                          n130 = Concatenate Strings(w526, w525, "_Corr_ToBeDeleted_", w528) -> (w523:string)
                          n131 = call "SetSpool_WaitForExtTrigger.vi"("path and name"=w523, "Kinetic Series"=w527) -> ()  [unwired: 10 in]
                        }
                        frame #2 {
                          # "groundtruth command"
                          # "response time of mirror"
                          n132 = call <userlib>:"LVClass_WavefrontCorrector Move to Absolute Position.vi"("WavefrontCorrector in"=w534, "Absolute Positions"=w533, "error in (no error)"=w532) -> ("error out"=w531:errorcluster)  [unwired: 11 in, 1 out]
                          n133 = Add(x=5, y=10) -> (x+y=w535:i32)
                          n134 = Wait (ms)(milliseconds to wait=w535) -> ()  [unwired: 1 out]
                        }
                        frame #3 {
                          # "take offset/groundtruth picture, only one"
                          n135 = local read "EMCCD trigger port"() -> (w539:tag)
                          n136 = call "trig EMCCD.vi"("error in (no error)"=w538, "exp time (ms)"=w542, "lines"=w539) -> ("error out"=w540:errorcluster)
                        }
                        frame #4 {
                          # "aberrated picture command"
                          # "response time of mirror"
                          n137 = call <userlib>:"LVClass_WavefrontCorrector Move to Absolute Position.vi"("WavefrontCorrector in"=w546, "Absolute Positions"=w545, "error in (no error)"=w544) -> ("error out"=w543:errorcluster)  [unwired: 11 in, 1 out]
                          n138 = Add(x=5, y=10) -> (x+y=w547:i32)
                          n139 = Wait (ms)(milliseconds to wait=w547) -> ()  [unwired: 1 out]
                        }
                        frame #5 {
                          # "take offset+initial aberr picture, only one"
                          n140 = local read "EMCCD trigger port"() -> (w551:tag)
                          n141 = call "trig EMCCD.vi"("error in (no error)"=w550, "exp time (ms)"=w552, "lines"=w551) -> ()  [unwired: 1 out]
                        }
                        frame #6 {
                          w568 = 1
                          # "correction command"
                          # "response time of mirror"
                          n142 = call-poly <vilib>:"Ramp Pattern.vi"("start"=w568, "end"=32, "delta"=w568) -> ("Ramp Pattern"=w566:dbl[])  [unwired: 6 in, 2 out]
                          n143 = call "zern2command_test.vi"("Initial haso file"=w553, "error in (no error)"=w561, "interaction matrix file"=w564, "Zern coef in"=w565, "Zern index in"=w566) -> ("error out"=w556:errorcluster, "Offset positions"=w562:sgl[])  [unwired: 4 in, 1 out]
                          n144 = Add(x=w563, y=w562) -> (x+y=w554:dbl[])
                          n145 = call <userlib>:"LVClass_WavefrontCorrector Move to Absolute Position.vi"("WavefrontCorrector in"=w557, "Absolute Positions"=w554, "error in (no error)"=w556) -> ("error out"=w555:errorcluster)  [unwired: 11 in, 1 out]
                          n146 = Add(x=5, y=10) -> (x+y=w558:i32)
                          n147 = Wait (ms)(milliseconds to wait=w558) -> ()  [unwired: 1 out]
                        }
                        frame #7 {
                          # "corrected pictures"
                          n148 = for {
                            N: w571 -> [_]
                            tunnel: w572 -> [w575]
                            shift-right: [w573] -> w569
                            shift-left: w570 -> [w574]
                            n149 = local read "EMCCD trigger port"() -> (w576:tag)
                            n150 = call "trig EMCCD.vi"("error in (no error)"=w574, "exp time (ms)"=w575, "lines"=w576) -> ("error out"=w573:errorcluster)
                          }
                        }
                        frame #8 {
                          # "one more trigger to end picture acquisition"
                          n151 = local read "EMCCD trigger port"() -> (w577:tag)
                          n152 = call "trig EMCCD.vi"("exp time (ms)"=w578, "lines"=w577) -> ()  [unwired: 1 in, 1 out]
                        }
                        frame #9 {
                          w585 = 0
                          # "save:\none groundtruth picture\none offset+abrr picture\nPictures per phase*corrected picture"
                          n153 = Number To Fractional String(number=w582, precision (6)=w585) -> (F-format string=w584:string)  [unwired: 2 in]
                          n154 = Concatenate Strings(w580, "_grdtrth_abrr_Corr_", w584, ".tif") -> (w589:string)
                          "Corrected Picture name" <- w589
                          n155 = Concatenate Strings(w581, w589) -> (w583:string)
                          n156 = call <userlib>:"SaveAsTiff.vi"("path"=w583, "palette"="C:\\Program Files\\Andor SOLIS\\GREY.PAL", "position"=w585, "type"=1) -> ()  [unwired: 10 in, 2 out]
                        }
                        frame #10 {
                          n157 = case shown="True" TRUE {
                            tunnel: w592 -> [_ w594]
                            tunnel: w590 -> [_ w593]
                            frame False {
                            }
                            frame True {
                              # "delete spooling data"
                              n158 = for {
                                N: w593 -> [_]
                                tunnel: w594 -> [w601]
                                i -> [w599]
                                n159 = Number To Fractional String(number=w599, precision (6)=0) -> (F-format string=w597:string)  [unwired: 2 in]
                                n160 = Concatenate Strings(w601, "000000000", w597, ".dat") -> (w596:string)
                                n161 = String To Path(string=w596) -> (path=w602:path)
                                n162 = Delete(path (use dialog)=w602) -> ()  [unwired: 4 in, 3 out]
                              }
                            }
                          }
                        }
                      }
                    }
                  }
                }
                frame #8 {
                  # "delete spooling data of phase diversity"
                  n163 = case shown="True" TRUE {
                    tunnel: w605 -> [_ w607]
                    tunnel: w603 -> [_ w606]
                    frame False {
                    }
                    frame True {
                      n164 = for {
                        N: w606 -> [_]
                        tunnel: w607 -> [w610]
                        i -> [w609]
                        n165 = Number To Fractional String(number=w609, precision (6)=0) -> (F-format string=w612:string)  [unwired: 2 in]
                        n166 = Concatenate Strings(w610, "000000000", w612, ".dat") -> (w608:string)
                        n167 = String To Path(string=w608) -> (path=w615:path)
                        n168 = Delete(path (use dialog)=w615) -> ()  [unwired: 4 in, 3 out]
                      }
                    }
                  }
                }
              }
            }
          }
          frame #3 {
            # "shut down shutter of 488nm laser"
            n169 = invoke class="MG17Motor" method="SC_Disable"(reference=w619, "lChanID"=w618) -> (reference out=w617:refnum<k7>, "lChanID"=w616:i32)  [unwired: 2 in, 2 out]
          }
          frame #4 {
            # "save the RMS of (calculated zer-real zer)"
            n170 = Concatenate Strings(w622, w621, "_RMSE.txt") -> (w627:string)
            n171 = String To Path(string=w627) -> (path=w626:path)
            n172 = Number To Fractional String(number=w623) -> (F-format string=w624:string[])  [unwired: 3 in]
            n173 = Write to Text File(file (use dialog)=w626, text=w624) -> (error out=w620:errorcluster)  [unwired: 2 in, 2 out]
          }
        }
        n174 = Merge Errors(w181, w180, w175) -> (w174:errorcluster)
        "Error out" <- w174
        n175 = Unbundle(w174) -> ("status"=w170:bool)  [unwired: 2 out]
        n176 = case shown="True" w170 {
          tunnel: [w196 w197] -> w173
          tunnel: w170 -> [w195 w197]
          frame False {
            n177 = Not(x=w195) -> (.not. x?=w196:bool)
          }
          frame True {
          }
        }
        n178 = Or(x=w173, y="?") -> (x .or. y?=w171:bool)
      }
    }
    frame #4 {
      # "# of z slices"
      # "open 488 shutter\napply correction matrix to DM\nset spooling\ntake picture from Z_top to Z_bottom in a step of delta_Z, show current Z\nall these pictures in one .tif file\nturn off shutter"
      n179 = Multiply(x="Z scanning range (um)", y=2.0) -> (x*y=w635:dbl)
      n180 = Divide(x=w635, y="Z scanning step (um)") -> (x/y=w634:dbl)
      n181 = Increment(x=w634) -> (x+1=w633:dbl)
      n182 = stacked-sequence {
        seq-local: [w642 _ _ _ _ _ _ _] -> [_ _ _ _ _ _ _ _]
        seq-local: [w641 _ _ _ _ _ _ _] -> [_ _ _ _ _ _ _ _]
        tunnel: w640 -> [w644 _ _ _ _ _ _ w711]
        tunnel: w639 -> [w643 _ _ _ _ _ _ w710]
        tunnel: w638 -> [_ w646 _ _ _ _ _ _]
        tunnel: w637 -> [_ w645 _ _ _ _ _ _]
        tunnel: w633 -> [_ _ w649 w655 _ _ w692 _]
        tunnel: w632 -> [_ _ w648 _ _ w686 w691 _]
        tunnel: w631 -> [_ _ w647 _ _ w685 w690 _]
        tunnel: "Z scanning range (um)" -> [_ _ _ w653 _ _ _ _]
        tunnel: "Z scanning step (um)" -> [_ _ _ w654 _ _ _ _]
        tunnel: w628 -> [_ _ _ w652 w681 _ _ _]
        frame #0 {
          n183 = invoke class="MG17Motor" method="SC_Enable"(reference=w644, "lChanID"=w643) -> (reference out=w642:refnum<k7>, "lChanID"=w641:i32)  [unwired: 2 in, 2 out]
        }
        frame #1 {
          n184 = call <userlib>:"LVClass_WavefrontCorrector Move to Absolute Position.vi"("WavefrontCorrector in"=w645, "Absolute Positions"=w646) -> ()  [unwired: 12 in, 2 out]
        }
        frame #2 {
          n185 = Concatenate Strings(w648, w647, "_3D") -> (w650:string)
          n186 = call "SetSpool_WaitForExtTrigger.vi"("path and name"=w650, "Kinetic Series"=w649) -> ()  [unwired: 10 in]
        }
        frame #3 {
          n187 = for {
            N: w655 -> [_]
            tunnel: w654 -> [w659]
            tunnel: w653 -> [w658]
            tunnel: w652 -> [w657]
            i -> [w656]
            n188 = stacked-sequence {
              tunnel: w659 -> [w664 _ _ _]
              tunnel: w658 -> [w667 _ _ _]
              tunnel: w657 -> [_ _ _ w679]
              tunnel: w656 -> [w665 _ _ _]
              frame #0 {
                # "10 step=1um"
                # "move to z"
                n189 = local read "Z for correction (um) (10 steps=1um)"() -> (w668:dbl)
                n190 = local read "ASI stage VISA resource name"() -> (w669:refnum<visa-resource-name>)
                n191 = Subtract(x=w668, y=w667) -> (x-y=w666:dbl)
                n192 = Multiply(x=w664, y=w665) -> (x*y=w663:dbl)
                n193 = Add(x=w666, y=w663) -> (x+y=w662:dbl)
                n194 = Multiply(x=w662, y=10) -> (x*y=w660:dbl)
                n195 = Number To Decimal String(number=w660) -> (decimal integer string=w671:string)  [unwired: 1 in]
                n196 = Concatenate Strings("move z=", w671) -> (w670:string)
                n197 = call "WriteCmd.vi"("Command"=w670, "VISA resource name"=w669) -> ()  [unwired: 1 in, 1 out]
              }
              frame #1 {
                n198 = Wait (ms)(milliseconds to wait=300) -> ()  [unwired: 1 out]
              }
              frame #2 {
                # "show z coordinate"
                n199 = local read "ASI stage VISA resource name"() -> (w677:refnum<visa-resource-name>)
                n200 = call "WriteCmd.vi"("Command"="where z", "VISA resource name"=w677) -> ("error"=w678:errorcluster)  [unwired: 1 in]
                n201 = VISA Read(VISA resource name=w677, byte count=100, error in (no error)=w678) -> (read buffer=→"Current Z in step":string)  [unwired: 3 out]
              }
              frame #3 {
                # "send a trigger to take picture"
                n202 = local read "EMCCD trigger port"() -> (w680:tag)
                n203 = call "trig EMCCD.vi"("exp time (ms)"=w679, "lines"=w680) -> ()  [unwired: 1 in, 1 out]
              }
            }
          }
        }
        frame #4 {
          # "send a trigger to end the acquisition"
          n204 = local read "EMCCD trigger port"() -> (w682:tag)
          n205 = call "trig EMCCD.vi"("exp time (ms)"=w681, "lines"=w682) -> ()  [unwired: 1 in, 1 out]
        }
        frame #5 {
          # "save .tif"
          n206 = Concatenate Strings(w686, w685, "_3D.tif") -> (w683:string)
          n207 = call <userlib>:"SaveAsTiff.vi"("path"=w683, "palette"="C:\\Program Files\\Andor SOLIS\\GREY.PAL", "position"=0, "type"=1) -> ()  [unwired: 10 in, 2 out]
        }
        frame #6 {
          # "delete spooling data"
          n208 = for {
            N: w692 -> [_]
            tunnel: w691 -> [w701]
            tunnel: w690 -> [w700]
            i -> [w693]
            n209 = Number To Decimal String(number=w693) -> (decimal integer string=w699:string)  [unwired: 1 in]
            n210 = String Length(string=w699) -> (length=w697:i32)
            n211 = Subtract(x=10, y=w697) -> (x-y=w696:i32)
            n212 = for {
              N: w696 -> [_]
              shift-right: [w709] -> w694
              shift-left: "_3D" -> [w708]
              n213 = Concatenate Strings(w708, "0") -> (w709:string)
            }
            n214 = Number To Fractional String(number=w693, precision (6)=0) -> (F-format string=w704:string)  [unwired: 2 in]
            n215 = Concatenate Strings(w701, w700, w694, w704, ".dat") -> (w702:string)
            n216 = String To Path(string=w702) -> (path=w706:path)
            n217 = Delete(path (use dialog)=w706) -> ()  [unwired: 4 in, 3 out]
          }
        }
        frame #7 {
          # "488 shutter off"
          n218 = invoke class="MG17Motor" method="SC_Disable"(reference=w711, "lChanID"=w710) -> ()  [unwired: 2 in, 4 out]
        }
      }
    }
    frame #5 {
      n219 = case shown="True" "Turn off EMCCD when finished?" {
        frame False {
        }
        frame True {
          n220 = flat-sequence {
            frame #0 {
              n221 = call <userlib>:"CoolerOFF.vi"() -> ()  [unwired: 2 in, 2 out]
            }
            frame #1 {
              # "shut down EMCCD"
              n222 = call <userlib>:"ShutDown.vi"() -> ()  [unwired: 2 in, 2 out]
            }
          }
        }
      }
    }
    frame #6 {
      # "shut down casao"
      n223 = call <userlib>:"LVClass_WavefrontCorrector dtor.vi"("WavefrontCorrector in"=w716, "error in (no error)"=w714) -> ("error out"=w713:errorcluster)  [unwired: 12 in, 1 out]
      n224 = call <userlib>:"LVClass_WavefrontCorrectorSet dtor.vi"("WavefrontCorrectorSet in"=w715, "error in (no error)"=w713) -> ()  [unwired: 12 in, 2 out]
      n225 = invoke class="MG17Motor" method="StopCtrl"(reference=w717) -> ()  [unwired: 2 in, 3 out]
    }
  }
